vi "TIO Data Stream Parse dstream Info.vi"(8 "dstreams in":T1(array[cluster]), 11 "dstream info raw":string="\u0000\u0000\u0001\u0000\b\u0000\u0000\u0000\u0000\u0000\u0000\u0000\u0006Ô\u0010\u0000\u0000\u0000\u0000\u0000\u0005\u0000\u0000\u0000\u0005\u0000\u0001\u0000\u0000\u0000\u0000\u0000\u0001\u0000\u0000\u0000\u0000\u0000\u0000\u0000\u0001\u0000\u0000\u0000\u0005\u0000\u0000\u0000\u0000\u0000\u0000\u0000\u0002\u0000\u0000\u0000\u0005\u0000\u0000\u0000\u0000\u0000\u0000\u0000\u0003\u0000\u0000\u0000d\u0000\u0000\u0000\u0000\u0000\u0000\u0000\u0004\u0000\u0000\u0000d\u0000\u0000\u0000\u0000\u0000\u0000\u0000") -> (0 "dstreams in":T1(array[cluster]), 2 "dstream info":T2)   [LabVIEW 2019]
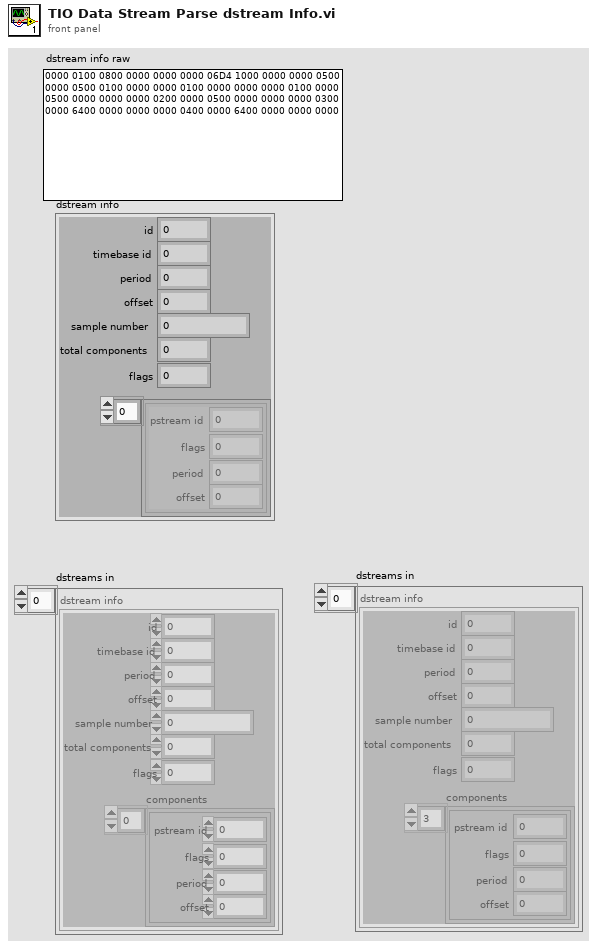
[diagram p1: front panel]
types:
  T1 = cluster{"id":u16, "timebase id":u16, "period":u32, "offset":u32, "sample number":u64, "total components":u16, "flags":u16, "components":cluster{"pstream id":u16, "flags":u16, "period":u32, "offset":u32}[]}[]
  T2 = cluster{"id":u16, "timebase id":u16, "period":u32, "offset":u32, "sample number":u64, "total components":u16, "flags":u16, cluster{"pstream id":u16, "flags":u16, "period":u32, "offset":u32}[]}
  T3 = enum16{"big-endian, network order", "native, host order", "little-endian"}
  T4 = cluster{"u16":u16, "u16":u16, "u32":u32, "u32":u32}
  T5 = cluster{"u16":u16, "u16":u16, "u32":u32, "u32":u32, "u64":u64, "u16":u16, "u16":u16}
  T6 = cluster{"id":u16, "timebase id":u16, "period":u32, "offset":u32, "sample number":u64, "total components":u16, "flags":u16, "components":cluster{"pstream id":u16, "flags":u16, "period":u32, "offset":u32}[]}
  T7 = cluster{"u16":u16, "u16":u16, "u32":u32, "u32":u32, "u64":u64, "u16":u16, "u16":u16, cluster{"u16":u16, "u16":u16, "u32":u32, "u32":u32}[]}
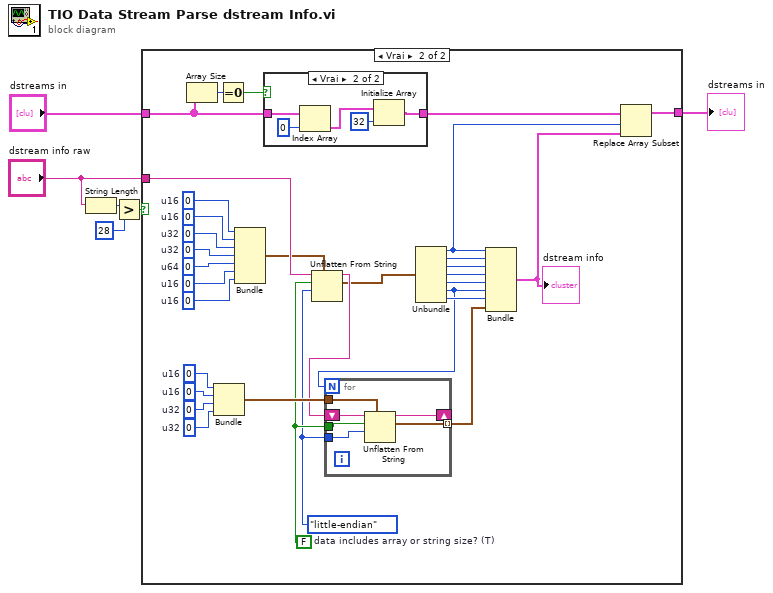
[diagram p0: block diagram]
diagram:
  n1 = String Length(string="dstream info raw") -> (length=w5:i32)
  n2 = Greater?(x=w5, y=28) -> (0:w4:bool)
  n3 = case shown="Vrai" w4 {
    tunnel: "dstream info raw" -> [_ w39]
    tunnel: "dstreams in" -> [w7 w13]
    tunnel: [w7 w10] -> w1
    frame False {
    }
    frame True {
      w25 = u16 0  # u16
      w26 = u16 0  # u16
      w27 = u64 0  # u64
      w28 = u32 0  # u32
      w29 = u32 0  # u32
      w30 = u16 0  # u16
      w31 = u16 0  # u16
      w35 = u32 0  # u32
      w36 = u32 0  # u32
      w37 = u16 0  # u16
      w38 = u16 0  # u16
      w33 = FALSE  # data includes array or string size? (T)
      w32 = T3."little-endian" ("byte order (0:big-endian, network order)")
      n4 = Array Size(array=w13) -> (size(s)=w15:i32)
      n5 = Bundle("u16"=w38, "u16"=w37, "u32"=w36, "u32"=w35) -> (w34:T4)  [unwired: 1 in]
      n6 = Equal To 0?(x=w15) -> (x = 0?=w14:bool)
      n7 = Bundle("u16"=w31, "u16"=w30, "u32"=w29, "u32"=w28, "u64"=w27, "u16"=w26, "u16"=w25) -> (w24:T5)  [unwired: 1 in]
      n8 = case shown="Vrai" w14 {
        tunnel: [w40 w45] -> w11
        tunnel: w13 -> [w40 w43]
        frame False {
        }
        frame True {
          n9 = Index Array(array=w43, index=0) -> (element=w41:T6)
          n10 = Initialize Array(w41, 32 ("dimension size")) -> (w45:T1)
        }
      }
      n11 = Unflatten From String(type=w24, binary string=w39, data includes array or string size? (T)=w33, byte order (0:big-endian, network order)=w32) -> (rest of the binary string=w23:string, value=w22:T5)  [unwired: 1 in, 1 out]
      n12 = Unbundle(w22) -> ("u16"=w9:u16, "u16"=w21:u16, "u32"=w20:u32, "u32"=w19:u32, "u64"=w18:u64, "u16"=w16:u16, "u16"=w17:u16)
      n13 = for {
        N: w16 -> [_]
        tunnel: w34 -> [w51]
        tunnel: w32 -> [w50]
        tunnel: w33 -> [w49]
        tunnel: [w47] -> w12 mode=indexing
        shift-right: [w46] -> _
        shift-left: w23 -> [w48]
        n14 = Unflatten From String(type=w51, binary string=w48, data includes array or string size? (T)=w49, byte order (0:big-endian, network order)=w50) -> (rest of the binary string=w46:string, value=w47:T4)  [unwired: 1 in, 1 out]
      }
      n15 = Bundle("u16"=w9, "u16"=w21, "u32"=w20, "u32"=w19, "u64"=w18, "u16"=w16, "u16"=w17, w12) -> (w8:T7)  [unwired: 1 in]
      "dstream info" <- w8
      n16 = Replace Array Subset(array=w11, new element=w8, index=w9) -> (w10:T1)
    }
  }
  "dstreams in" <- w1
